vi "Set protocol data.vi"(7 "Operation":T1, 8 "error in (no error)":errorcluster, 10 "Protocols.lvlib:Protocol Parent.lvclass":refnum<class "Protocol Parent.lvclass">, 11 "Listener In.lvclass":refnum<class "Listener.lvclass"> caption="Listener") -> (0 "error out":errorcluster, 3 "Listener Out.lvclass":refnum<class "Listener.lvclass">)   [LabVIEW 2019, in "Listener.lvclass"]
uses:
  Listener.lvclass
  Protocol Parent/Protocol Parent.lvclass
  ListenerClassControls/Operation.ctl
  AK TCP/AK TCP.lvclass
  D:/GitRepository/niveristand-instrument-addon-classes/Source/Protocols/TCP/TCP.lvclass
  ListenerClassControls/AK TCP Data Structure.ctl
  ListenerClassControls/Protocol.ctl
  TCP/TCP.lvclass/TCP.ctl
  TCP/TCP.lvclass
  ListenerClassControls/TCP Data Structure.ctl
  UDP/UDP.lvclass
  ListenerClassControls/UDP Data Structure.ctl
  UDP/UDP.lvclass/UDP.ctl
  TCP/Data Access/Read IP Address.vi
  TCP/Data Access/Read Port.vi
  UDP/Data Access/Read Target IP Address.vi
  UDP/Data Access/Read Local Port.vi
  UDP/Data Access/Read Local IP Address.vi
  UDP/Data Access/Read Target Port.vi
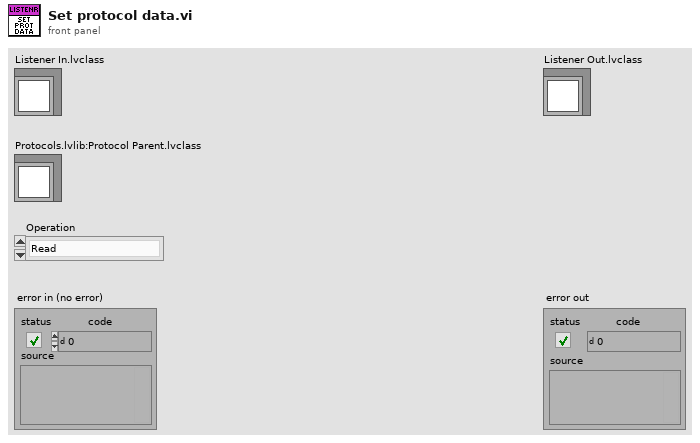
[diagram p1: front panel]
types:
  T1 = typedef "Listener.lvclass/Operation.ctl" = enum16{"Read", "Write"}
  T2 = typedef "Listener.lvclass/Protocol.ctl" = enum16{"RS-XXX", "AK RS-XXX", "VISA", "TCPIP", "AK TCPIP", "UDP", "GPIB ConvBox"}
  T3 = typedef "Listener.lvclass/AK TCP Data Structure.ctl" = cluster{"TCP|IP connection ID":refnum<k5>, "IP Address":string, "Port":u16, "Data":string, "Current Command Code":string}
  T4 = typedef "Listener.lvclass/TCP Data Structure.ctl" = cluster{"TCP|IP connection ID":refnum<k5>, "IP Address":string, "Port":u16, "Data":string}
  T5 = typedef "Listener.lvclass/UDP Data Structure.ctl" = cluster{"UDP connection ID":refnum<k16>, "Local Address":string, "Local Port":u16, "Target IP Address":string, "Target Port":u16, "Data":string}
  T6 = typedef "Protocols.lvlib/Protocol Parent.lvclass/Base Protocol Type.ctl" = enum16{"RS-XXX", "VISA", "TCPIP", "UDP", "GPIB ConvBox"}
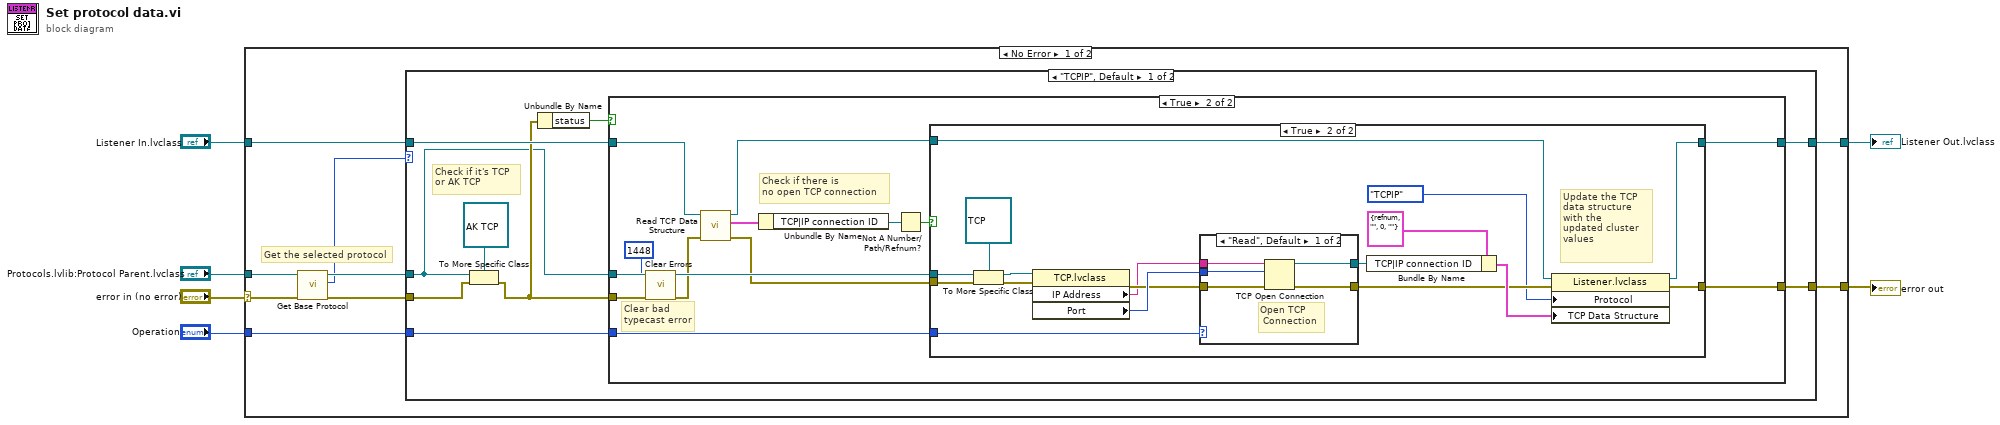
[diagram p0: block diagram]
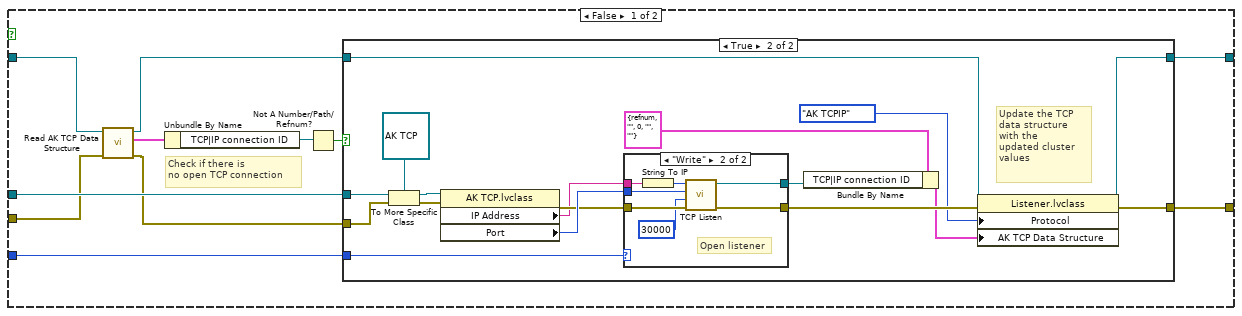
[diagram p2: hidden frame]
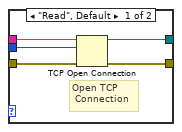
[diagram p4: hidden frame]
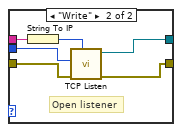
[diagram p6: hidden frame]
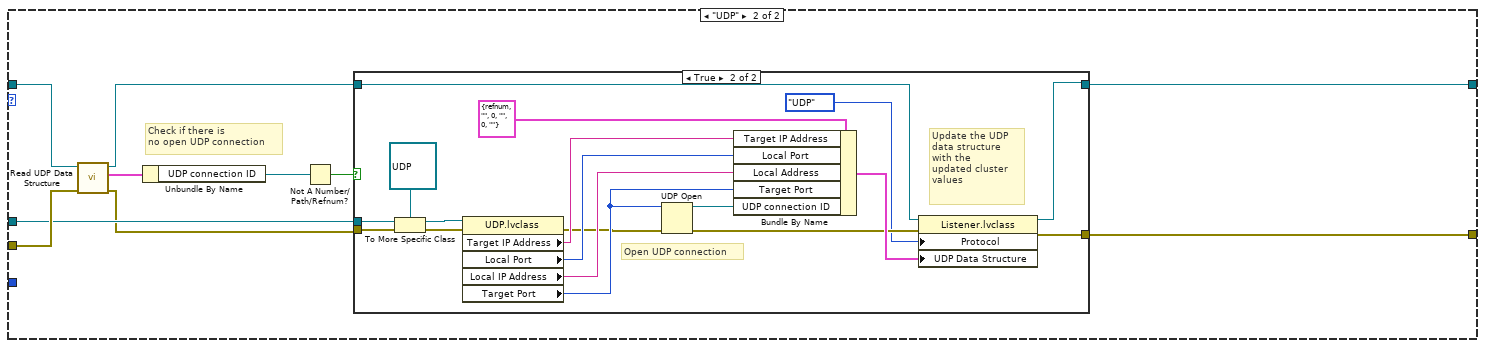
[diagram p7: hidden frame]
diagram:
  n1 = case shown="No Error" "error in (no error)" {
    selector: "error in (no error)" -> [w13 w141]
    tunnel: [w12 w141] -> w5
    tunnel: "Protocols.lvlib:Protocol Parent.lvclass" -> [w14 _]
    tunnel: "Listener In.lvclass" -> [w11 w140]
    tunnel: [w8 w140] -> w2
    tunnel: "Operation" -> [w7 _]
    frame No Error {
      # "Get the selected protocol"
      n2 = call-dynamic "Get Base Protocol.vi"("error in (no error)"=w13, "Protocol Parent in"=w14) -> ("error out"=w10:errorcluster, "Protocol out"=w9:T6, "Protocol Parent out"=w15:refnum<class "Protocol Parent.lvclass">)  [unwired: 7 in]
      n3 = case shown="\"TCPIP\", Default" w9 {
        tunnel: w15 -> [w16 w113]
        tunnel: w10 -> [w20 w115]
        tunnel: [w23 w118] -> w12
        tunnel: w11 -> [w22 w114]
        tunnel: [w24 w119] -> w8
        tunnel: w7 -> [w21 _]
        frame "TCPIP", Default {
          # "Check if it's TCP \nor AK TCP"
          n4 = To More Specific Class(target class=refnum<class "AK TCP.lvclass"> refnum ("Protocols.lvlib:AK TCP.lvclass"), reference=w16, error in=w20) -> (error out=w19:errorcluster)  [unwired: 1 out]
          n5 = Unbundle By Name(w19) -> ("status"=w18:bool)
          n6 = case shown="True" w18 {
            tunnel: w16 -> [w35 w79]
            tunnel: [w34 w78] -> w24
            tunnel: [w33 w77] -> w23
            tunnel: w22 -> [w30 w75]
            tunnel: w19 -> [w28 w74]
            tunnel: w21 -> [w31 w69]
            frame False {
              # "Check if there is \nno open TCP connection"
              n7 = call-dynamic "Read AK TCP Data Structure.vi"("error in (no error)"=w28, "Listener in"=w30) -> ("error out"=w27:errorcluster, "TCP|IP Data Structure"=w26:T3, "Listener out"=w29:refnum<class "Listener.lvclass">)  [unwired: 7 in]
              n8 = Unbundle By Name(w26) -> ("TCP|IP connection ID"=w25:refnum<k5>)
              n9 = Not A Number/Path/Refnum?(number/path/refnum=w25) -> (NaN/Path/Refnum?=w32:bool)
              n10 = case shown="True" w32 {
                tunnel: w35 -> [_ w54]
                tunnel: [w37 w51] -> w34
                tunnel: [w36 w50] -> w33
                tunnel: w27 -> [w36 w49]
                tunnel: w29 -> [w37 w48]
                tunnel: w31 -> [_ w47]
                frame False {
                }
                frame True {
                  # "Update the TCP \ndata structure\nwith the\nupdated cluster\nvalues"
                  n11 = To More Specific Class(target class=refnum<class "AK TCP.lvclass"> refnum ("Protocols.lvlib:AK TCP.lvclass"), reference=w54, error in=w49) -> (specific class reference=w53:refnum<class "AK TCP.lvclass">, error out=w52:errorcluster)
                  n12 = property class="AK TCP.lvclass"(reference=w53, error in=w52) -> (error out=w45:errorcluster, "IP Address"=w44:string, "Port"=w46:u16)  [unwired: 1 out]
                  n13 = case shown="\"Write\"" w47 {
                    tunnel: w46 -> [w59 w61]
                    tunnel: w45 -> [w58 w66]
                    tunnel: w44 -> [w57 w65]
                    tunnel: [w56 w62] -> w43
                    tunnel: [w55 w63] -> w42
                    frame "Read", Default {
                      # "Open TCP\n Connection"
                      n14 = TCP Open Connection(address=w57, remote port or service name=w59, error in (no error)=w58) -> (connection ID=w55:refnum<k5>, error out=w56:errorcluster)  [unwired: 2 in]
                    }
                    frame "Write" {
                      # "Open listener"
                      n15 = String To IP(1:w65) -> (0:w64:u32)
                      n16 = call <vilib>:"TCP Listen.vi"("net address"=w64, "error in (no error)"=w66, "timeout ms (wait forever: -1)"=30000, "port"=w61) -> ("error out"=w62:errorcluster, "connection ID"=w63:refnum<k5>)  [unwired: 3 in, 3 out]
                    }
                  }
                  n17 = Bundle By Name(cluster=T3 {"TCP|IP connection ID"=refnum, "IP Address"="", "Port"=0, "Data"="", "Current Command Code"=""} ("TCP|IP Data Structure"), "TCP|IP connection ID"=w42) -> (w39:T3)
                  n18 = property class="Listener.lvclass"(reference=w48, error in=w43, "Protocol"=Protocol."AK TCPIP", "AK TCP Data Structure"=w39) -> (reference out=w51:refnum<class "Listener.lvclass">, error out=w50:errorcluster)
                }
              }
            }
            frame True {
              # "Clear bad \ntypecast error"
              # "Check if there is \nno open TCP connection"
              n19 = call <vilib>:"Clear Errors.vi"("error in (no error)"=w74, "specific error code to clear (0: all)"=1448) -> ("error out"=w68:errorcluster)  [unwired: 4 in, 1 out]
              n20 = call-dynamic "Read TCP Data Structure.vi"("error in (no error)"=w68, "Listener in"=w75) -> ("error out"=w73:errorcluster, "TCP|IP Data Structure"=w72:T4, "Listener out"=w71:refnum<class "Listener.lvclass">)  [unwired: 7 in]
              n21 = Unbundle By Name(w72) -> ("TCP|IP connection ID"=w76:refnum<k5>)
              n22 = Not A Number/Path/Refnum?(number/path/refnum=w76) -> (NaN/Path/Refnum?=w70:bool)
              n23 = case shown="True" w70 {
                tunnel: w79 -> [_ w97]
                tunnel: [w81 w93] -> w78
                tunnel: [w80 w91] -> w77
                tunnel: w73 -> [w80 w90]
                tunnel: w71 -> [w81 w89]
                tunnel: w69 -> [_ w88]
                frame False {
                }
                frame True {
                  # "Update the TCP \ndata structure\nwith the\nupdated cluster\nvalues"
                  n24 = To More Specific Class(target class=refnum<class "TCP.lvclass"> refnum ("Protocols.lvlib:TCP.lvclass"), reference=w97, error in=w90) -> (specific class reference=w96:refnum<class "TCP.lvclass">, error out=w95:errorcluster)
                  n25 = property class="TCP.lvclass"(reference=w96, error in=w95) -> (error out=w86:errorcluster, "IP Address"=w85:string, "Port"=w87:u16)  [unwired: 1 out]
                  n26 = case shown="\"Read\", Default" w88 {
                    tunnel: w87 -> [w103 w108]
                    tunnel: w86 -> [w102 w109]
                    tunnel: w85 -> [w101 w107]
                    tunnel: [w100 w104] -> w84
                    tunnel: [w99 w105] -> w83
                    frame "Read", Default {
                      # "Open TCP\n Connection"
                      n27 = TCP Open Connection(address=w101, remote port or service name=w103, error in (no error)=w102) -> (connection ID=w99:refnum<k5>, error out=w100:errorcluster)  [unwired: 2 in]
                    }
                    frame "Write" {
                      # "Open listener"
                      n28 = String To IP(1:w107) -> (0:w106:u32)
                      n29 = call <vilib>:"TCP Listen.vi"("net address"=w106, "error in (no error)"=w109, "port"=w108) -> ("error out"=w104:errorcluster, "connection ID"=w105:refnum<k5>)  [unwired: 4 in, 3 out]
                    }
                  }
                  n30 = Bundle By Name(cluster=T4 {"TCP|IP connection ID"=refnum, "IP Address"="", "Port"=0, "Data"=""} ("TCP|IP Data Structure"), "TCP|IP connection ID"=w83) -> (w92:T4)
                  n31 = property class="Listener.lvclass"(reference=w89, error in=w84, "Protocol"=Protocol."TCPIP", "TCP Data Structure"=w92) -> (reference out=w93:refnum<class "Listener.lvclass">, error out=w91:errorcluster)
                }
              }
            }
          }
        }
        frame "UDP" {
          # "Check if there is \nno open UDP connection"
          n32 = call-dynamic "Read UDP Data Structure.vi"("error in (no error)"=w115, "Listener in"=w114) -> ("error out"=w111:errorcluster, "UDP Data Structure"=w112:T5, "Listener out"=w110:refnum<class "Listener.lvclass">)  [unwired: 7 in]
          n33 = Unbundle By Name(w112) -> ("UDP connection ID"=w116:refnum<k16>)
          n34 = Not A Number/Path/Refnum?(number/path/refnum=w116) -> (NaN/Path/Refnum?=w117:bool)
          n35 = case shown="True" w117 {
            tunnel: w111 -> [w121 w139]
            tunnel: w113 -> [_ w137]
            tunnel: w110 -> [w120 w131]
            tunnel: [w120 w130] -> w119
            tunnel: [w121 w128] -> w118
            frame False {
            }
            frame True {
              # "Update the UDP \ndata structure\nwith the\nupdated cluster\nvalues"
              # "Open UDP connection"
              n36 = To More Specific Class(target class=refnum<class "UDP.lvclass"> refnum ("Protocols.lvlib:UDP.lvclass"), reference=w137, error in=w139) -> (specific class reference=w127:refnum<class "UDP.lvclass">, error out=w136:errorcluster)
              n37 = property class="UDP.lvclass"(reference=w127, error in=w136) -> (error out=w125:errorcluster, "Target IP Address"=w135:string, "Local Port"=w134:u16, "Local IP Address"=w133:string, "Target Port"=w126:u16)  [unwired: 1 out]
              n38 = UDP Open(8:w125, 11:w126) -> (port=w124:refnum<k16>, 0:w123:errorcluster)  [unwired: 3 in, 1 out]
              n39 = Bundle By Name(cluster=T5 {"UDP connection ID"=refnum, "Local Address"="", "Local Port"=0, "Target IP Address"="", "Target Port"=0, "Data"=""} ("UDP Data Structure"), "Target IP Address"=w135, "Local Port"=w134, "Local Address"=w133, "Target Port"=w126, "UDP connection ID"=w124) -> (w129:T5)
              n40 = property class="Listener.lvclass"(reference=w131, error in=w123, "Protocol"=Protocol."UDP", "UDP Data Structure"=w129) -> (reference out=w130:refnum<class "Listener.lvclass">, error out=w128:errorcluster)
            }
          }
        }
      }
    }
    frame Error {
    }
  }
  "Listener Out.lvclass" <- w2
  "error out" <- w5
